vi "Get Paths Array UI.vi"(11 "Data":variant) -> (2 "Cancelled?":bool, 3 "selected_paths":string)   [LabVIEW 2019, in "LV-Data.PGSQL.lvclass"]
uses:
  LV-Data.PGSQL.lvclass
  Typedefs/Errors--enum.ctl
  <userlib>/_OpenG.lib/array/array.llb/Search 1D Array (String)__ogtk.vi
  <vilib>/regexp/Match Regular Expression.xnode
panel:
  in  "UNDO LAST VALUE":bool
  out "Paths":string[](array[string])
  out "Message":string
  out "path_to_selected_column":string="llab_038:d001(TEST_TABLE--new_stuff(hippos))"
  out "selected_table":string="TEST_TABLE"
  in  "columns_list":i32(listbox)=1
  in  "tables_list":i32(listbox)=34
  in  "STOP":bool
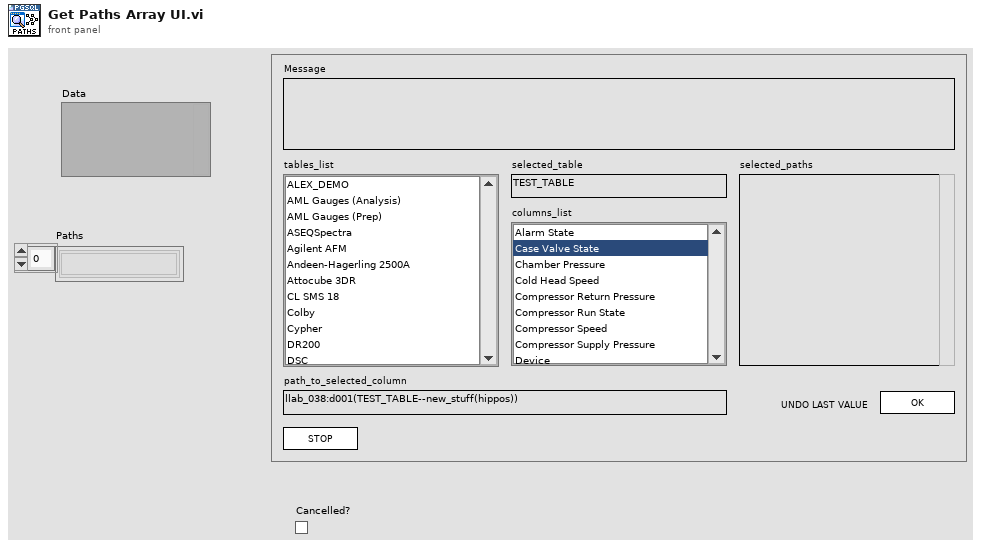
[diagram p1: front panel]
types:
  T1 = enum32{"Invalid", "Standard", "Closed", "Hidden", "Minimized", "Maximized"}
  T2 = enum32{"invalid app kind", "Development System", "Run Time System", "Student Edition", "Embedded LabVIEW", "Evaluation", "Custom"}
  T3 = enum32{"Bad", "Idle", "Run top level", "Running"}
  T4 = typedef "LV-Data.PGSQL.lvclass/Errors--enum.ctl" = enum16{"0: None", "5005: Path Type Not Supported", "5006: Number of Variables", "5007: Number of data points", "5008: Cannot write two data points", "5030: Start and End Times Identical", "5031: Input is not wholly", "5032: Undefined Timestamps", "5033: Bad path or paths", "5040: Invalid Instrument Name", "5050: Column can only hold string", "5051: Column can only hold bool", "5052: Column can only hold double", "5053: Column can only hold int"}
  T5 = cluster{"Core":cluster{"Current VI Reference":refnum<vi>, "Close Panel on Exit?":bool}, "Data.PG in":refnum<class "LV-Data.PGSQL.lvclass">, "table names":string[], "table paths":string[], "column names":string[], "column units":string[], "column paths":string[], "new table name":string, "new column name":string, "new column data type":string, "new column units":string, "selected table":string, "selected column":string, "selected table path":string, "selected column path":string, "selected column units":string, "Paths array":string[], "Current Index":i32, "Data":string[], "Type (Name)":string[]}
  T6 = cluster{"Current VI Reference":refnum<vi>, "Close Panel on Exit?":bool}
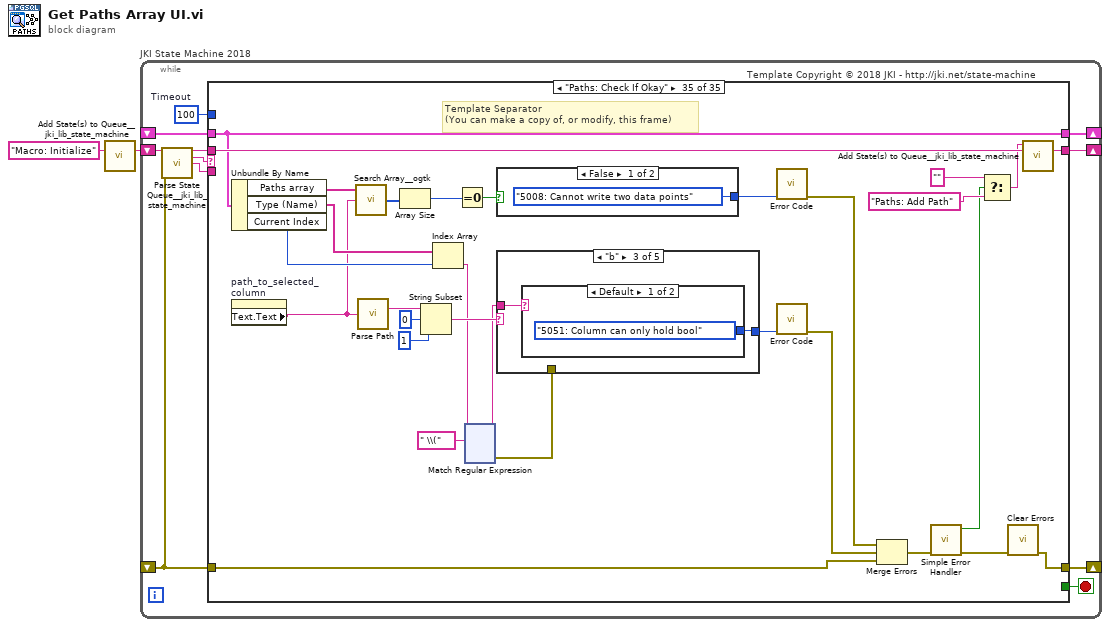
[diagram p0: block diagram]
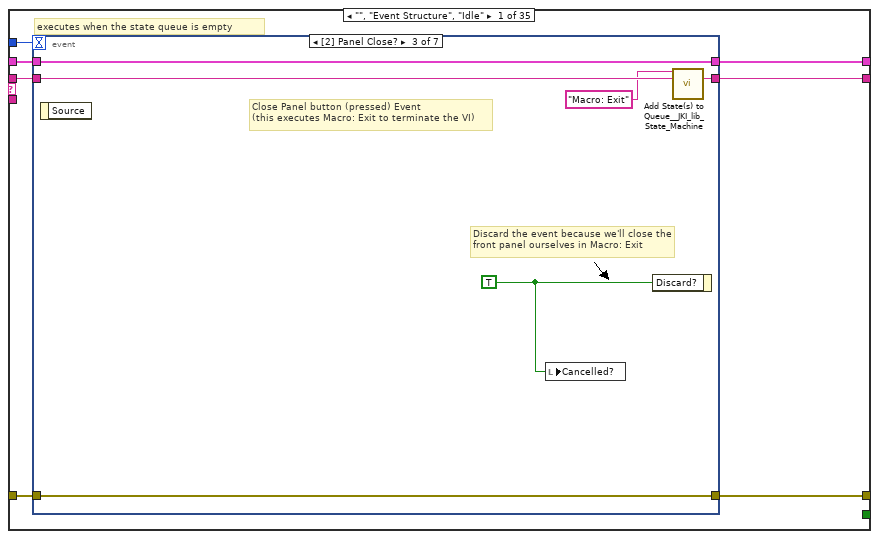
[diagram p2: hidden frame]
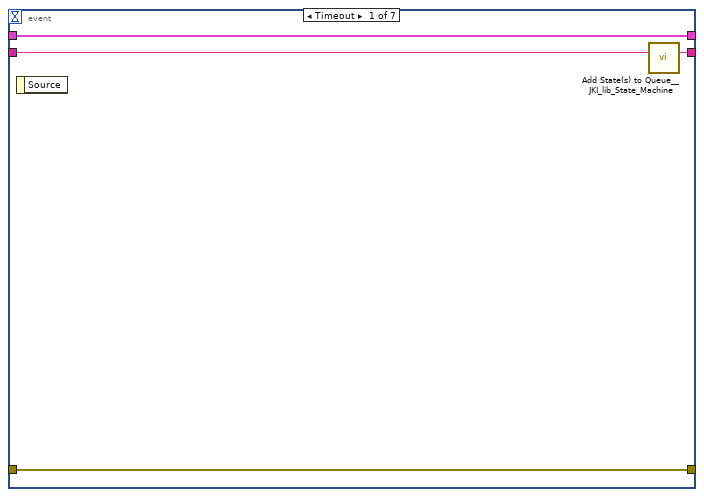
[diagram p3: hidden frame]
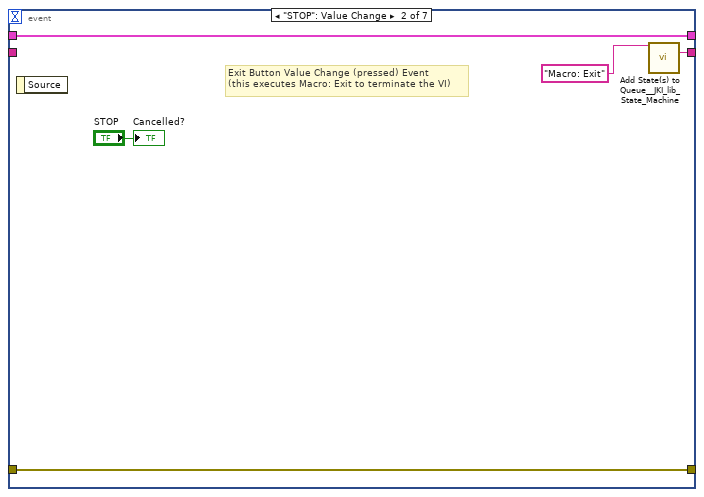
[diagram p4: hidden frame]
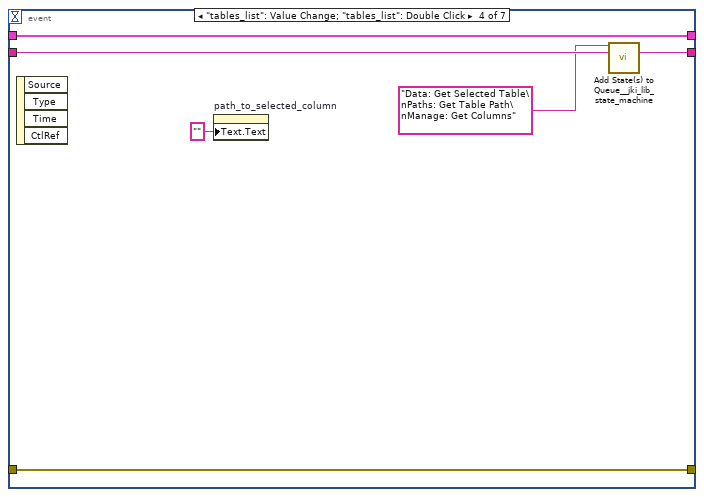
[diagram p5: hidden frame]
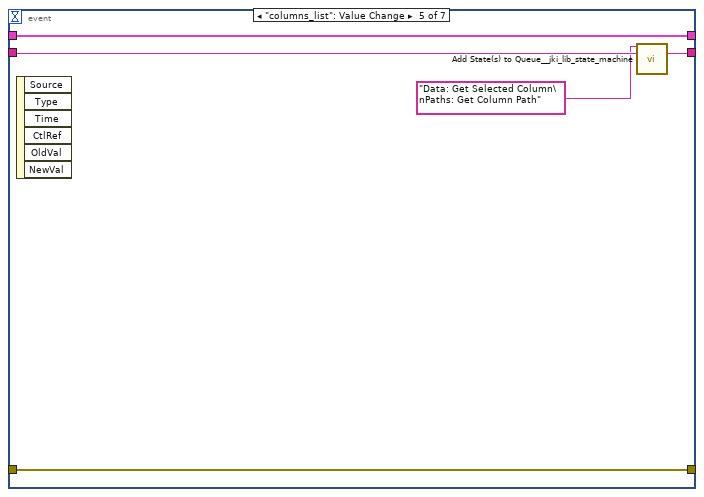
[diagram p6: hidden frame]
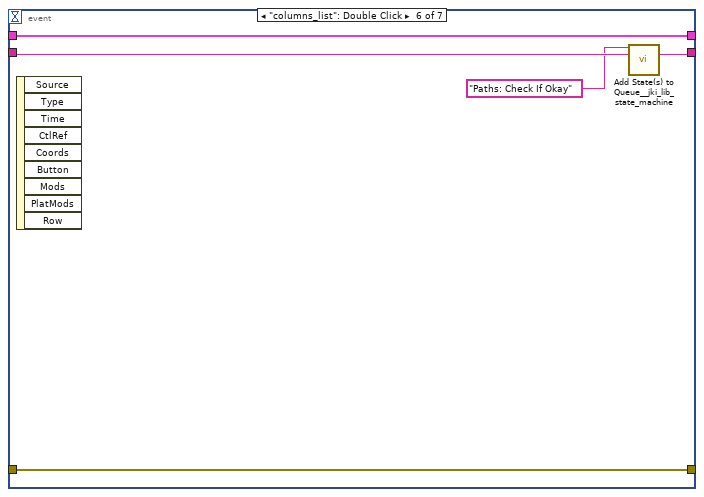
[diagram p7: hidden frame]
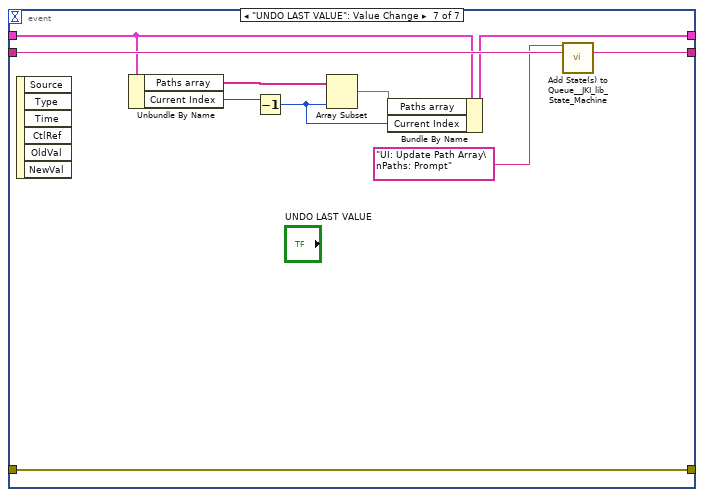
[diagram p8: hidden frame]
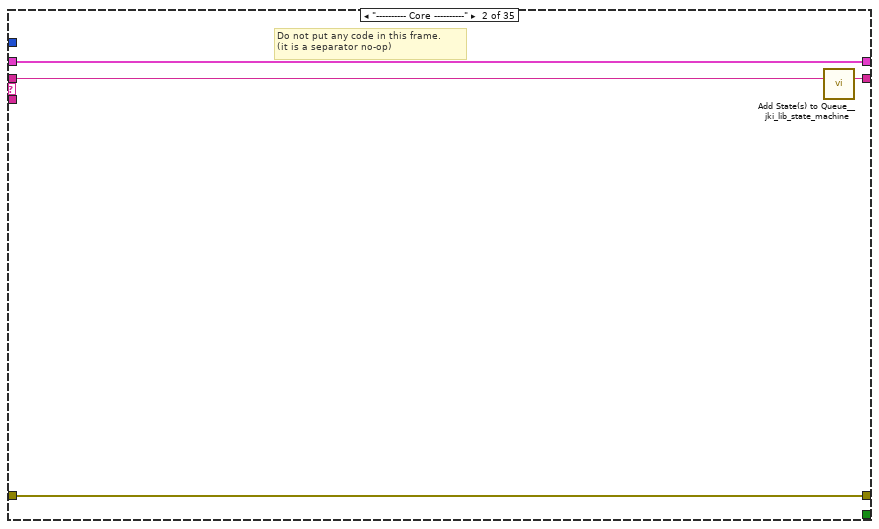
[diagram p9: hidden frame]
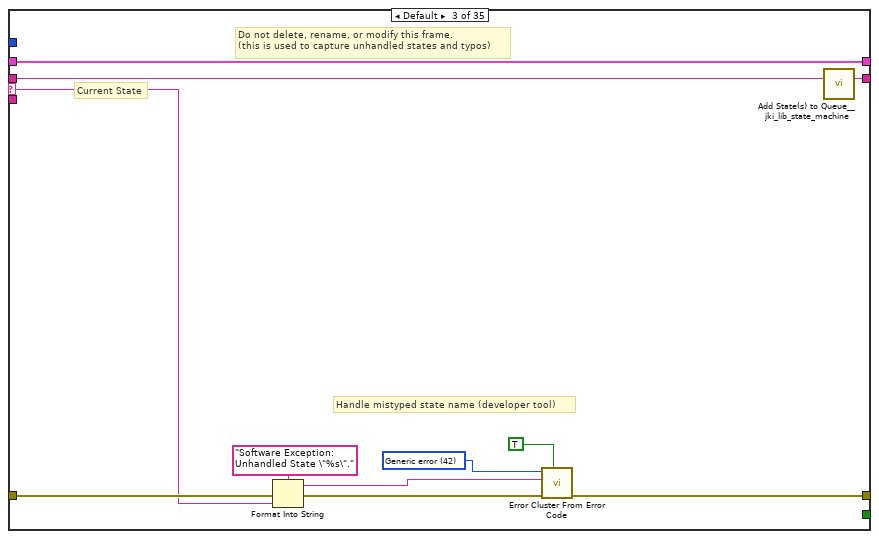
[diagram p10: hidden frame]
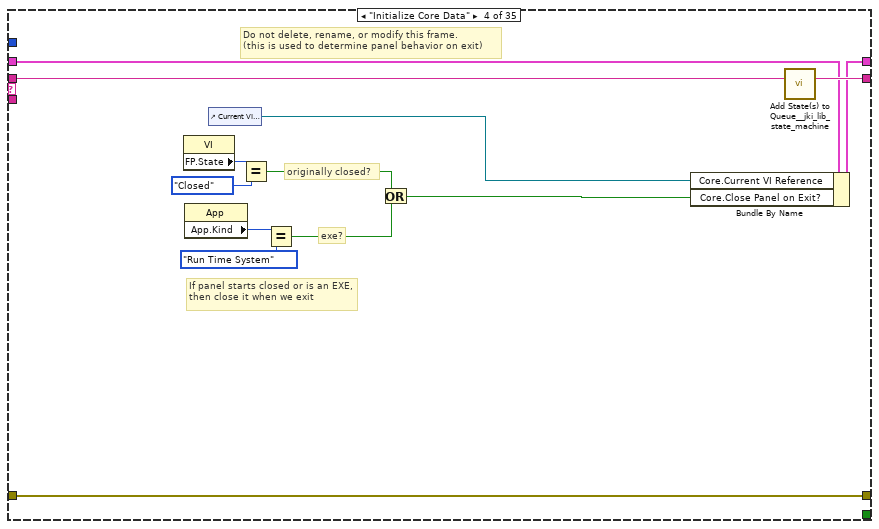
[diagram p11: hidden frame]
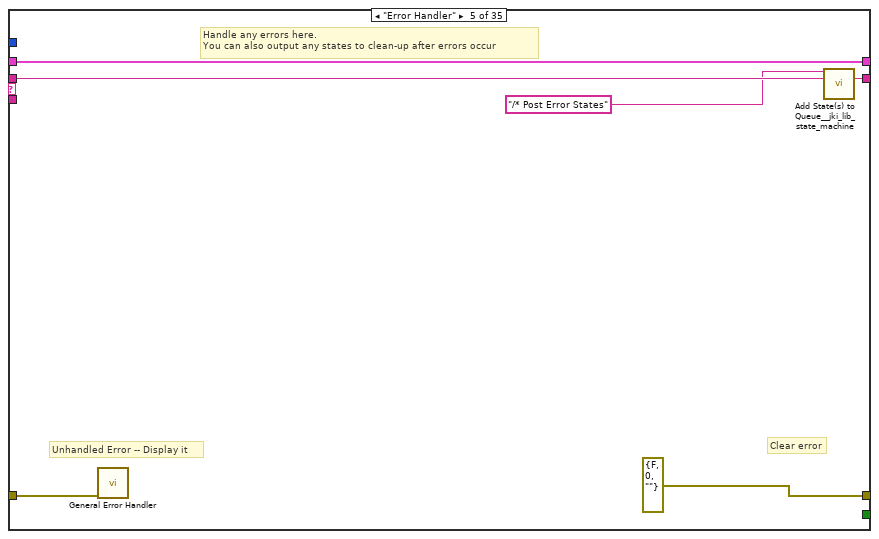
[diagram p12: hidden frame]
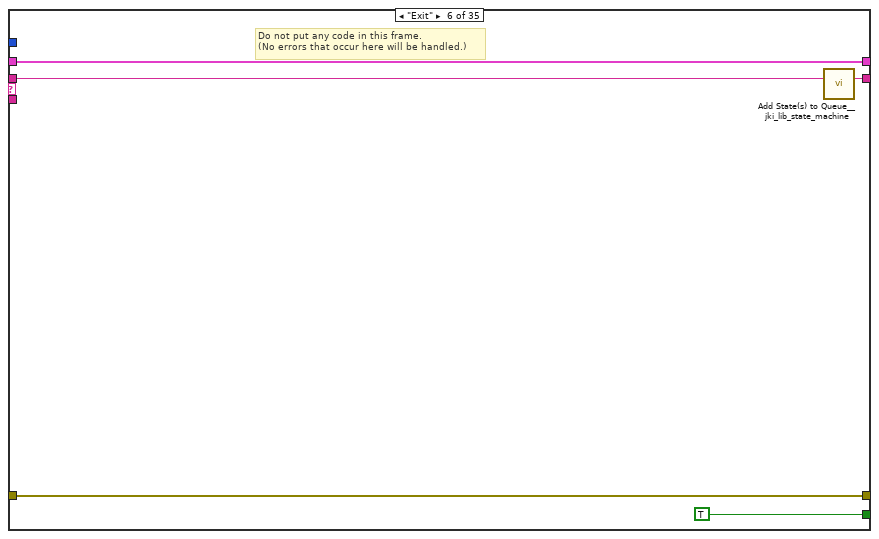
[diagram p13: hidden frame]
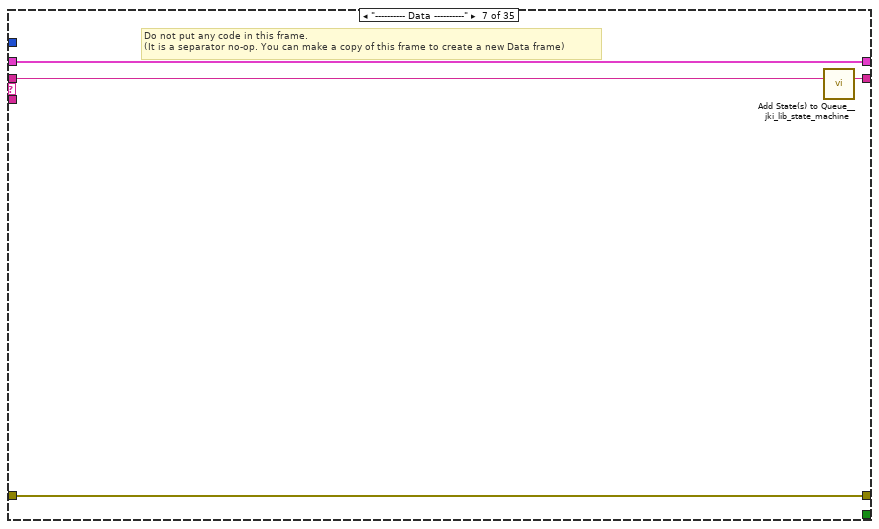
[diagram p14: hidden frame]
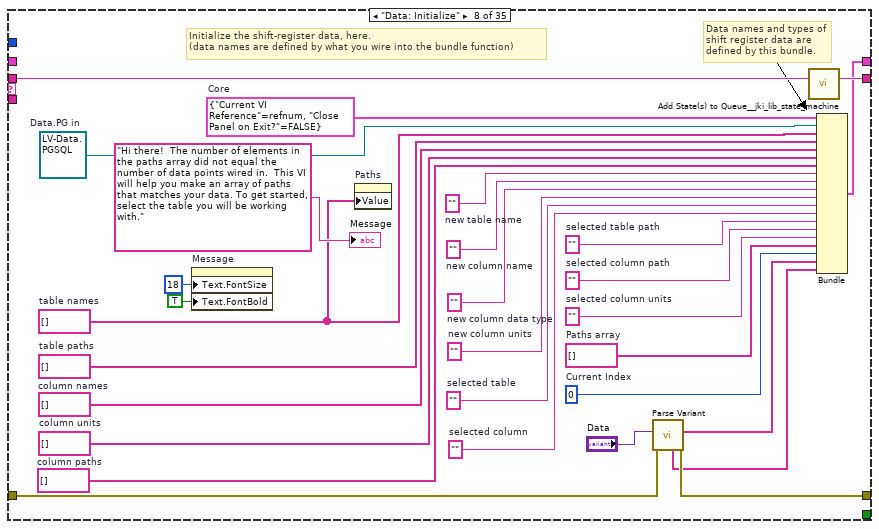
[diagram p15: hidden frame]
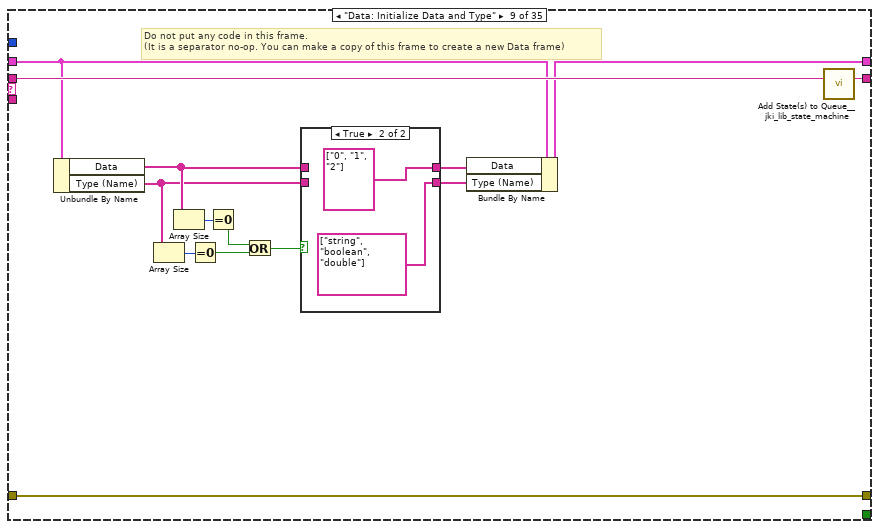
[diagram p16: hidden frame]
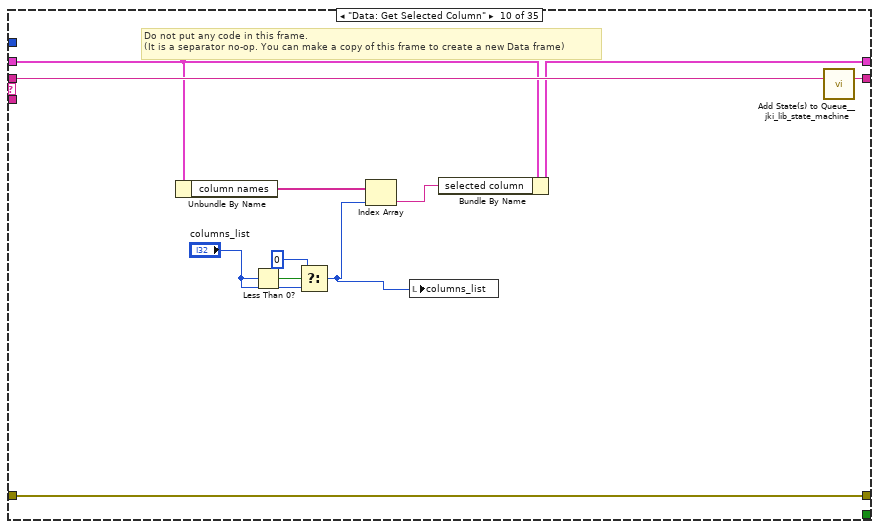
[diagram p18: hidden frame]
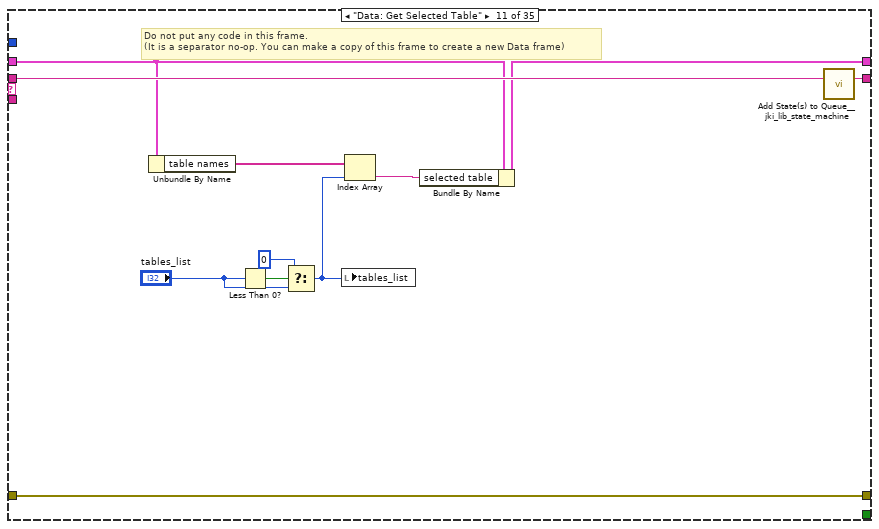
[diagram p19: hidden frame]
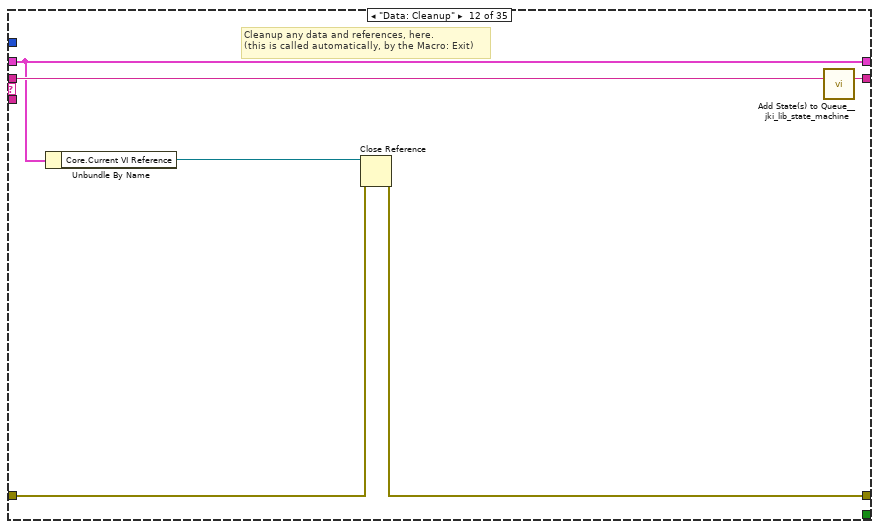
[diagram p20: hidden frame]
diagram:
  n1 = call <vilib>:"Add State(s) to Queue__jki_lib_state_machine.vi"("State(s) in (\"\")"="Macro: Initialize") -> ("States Out"=w2:string)  [unwired: 14 in]
  n2 = while "JKI State Machine 2018" {
    shift-right: [w6] -> _
    shift-left: _ -> [w5]
    shift-right: [w9] -> _
    shift-left: _ -> [w3]
    shift-right: [w8] -> _
    shift-left: w2 -> [w10]
    stop <- w7 stop-if-true
    w4 = 100  # Timeout
    # "Template Copyright © 2018 JKI - http://jki.net/state-machine"
    n3 = call <vilib>:"Parse State Queue__jki_lib_state_machine.vi"("State Queue"=w10, "Error In (no error)"=w3) -> ("Remaining States"=w12:string, "Current State"=w13:string, "Arguments"=w11:string)  [unwired: 11 in]
    n4 = case shown="\"Paths: Check If Okay\"" w13 {
      selector: w13 -> [_ _ w66 _ _ _ _ _ _ _ _ _ _ _ _ _ _ _ _ _ _ _ _ _ _ _ _ _ _ _ _ _ _ _ _]
      tunnel: w12 -> [w20 w65 w70 w89 w95 w100 w104 w133 w147 w162 w173 w179 w183 w194 w202 w208 w219 w291 w315 w323 w327 w332 w342 w346 w355 w368 w372 w378 w386 w390 w399 w413 w424 w443 w482]
      tunnel: w11 -> [_ _ _ _ _ _ _ _ _ _ _ _ _ _ _ w203 w213 _ w311 _ _ _ _ _ _ _ _ _ _ _ _ _ _ _ _]
      tunnel: w5 -> [w18 w62 w68 w82 w92 w98 w101 _ w144 w157 w168 w175 w180 w186 w197 w206 w215 w288 w312 w320 w324 w329 w339 w343 w353 w366 w369 w376 w384 w387 w397 w411 w421 w437 w480]
      tunnel: [w17 w63 w72 w86 errorcluster {"status"=FALSE, "code"=0, "source"=""} ("error out") w97 w102 w108 w145 w160 w171 w174 w181 w185 w200 w204 w216 w289 w313 w321 w325 w330 w340 w344 w349 w362 w370 w373 w380 w388 w393 w401 w422 w441 w465] -> w9
      tunnel: w3 -> [w16 w63 w71 w86 w91 w97 w102 w107 w145 w160 w171 w176 w181 w192 w200 w205 w217 w289 w313 w321 w325 w330 w340 w344 w350 w363 w370 w374 w381 w388 w394 w402 w422 w441 w462]
      tunnel: [w19 w64 w69 w88 w94 w99 w103 w132 w146 w161 w172 w178 w182 w193 w201 w207 w218 w290 w314 w322 w326 w331 w341 w345 w354 w367 w371 w377 w385 w389 w398 w412 w423 w442 w481] -> w8
      tunnel: [_ _ _ _ _ TRUE _ _ _ _ _ _ _ _ _ _ _ _ _ _ _ _ _ _ _ _ _ _ _ _ _ _ _ _ _] -> w7
      tunnel: [w15 w62 w68 w87 w92 w98 w101 w131 w143 w158 w167 w175 w180 w186 w197 w206 w215 w288 w312 w320 w324 w329 w339 w343 w352 w365 w369 w376 w383 w387 w391 w403 w421 w426 w480] -> w6
      tunnel: w4 -> [w14 _ _ _ _ _ _ _ _ _ _ _ _ _ _ _ _ _ _ _ _ _ _ _ _ _ _ _ _ _ _ _ _ _ _]
      frame "", "Event Structure", "Idle" {
        # "executes when the state queue is empty"
        n5 = event shown="[2] Panel Close?" {
          selector: _ -> [_ _ _ _ _ _ _]
          dyn-events: _ -> [_ _ _ _ _ _ _]
          timeout: w14 -> [_ _ _ _ _ _ _]
          tunnel: w20 -> [w24 _ w35 w39 w44 w49 w59]
          tunnel: [w23 w29 w34 w40 w45 w50 w60] -> w19
          tunnel: w18 -> [w21 w27 w32 w36 w46 w48 w56]
          tunnel: [w22 w28 w33 w41 w42 w51 w61] -> w17
          tunnel: w16 -> [w22 w28 w33 w41 w42 w51 w61]
          tunnel: [w21 w27 w32 w36 w46 w48 w55] -> w15
          event Timeout {
            n6 = event-data() -> ()  [unwired: 1 in, 1 out]
            n7 = call <vilib>:"Add State(s) to Queue__JKI_lib_State_Machine.vi"("State(s) in (\"\")"=w24) -> ("States Out"=w23:string)  [unwired: 14 in]
          }
          event "STOP": Value Change {
            # "Exit Button Value Change (pressed) Event\n(this executes Macro: Exit to terminate the VI)"
            n8 = event-data() -> ()  [unwired: 1 in, 1 out]
            n9 = call <vilib>:"Add State(s) to Queue__JKI_lib_State_Machine.vi"("State(s) in Front (\"\")"="Macro: Exit") -> ("States Out"=w29:string)  [unwired: 14 in]
            "Cancelled?" <- "STOP"
          }
          event Panel Close? {
            w30 = TRUE ("Discard?")
            # "Discard the event because we'll close the front panel ourselves in Macro: Exit"
            # "Close Panel button (pressed) Event\n(this executes Macro: Exit to terminate the VI)"
            n10 = event-data() -> ()  [unwired: 1 in, 1 out]
            n11 = local write "Cancelled?"(w30) -> ()
            n12 = event-data("Discard?"=w30) -> ()  [unwired: 1 in, 1 out]
            n13 = call <vilib>:"Add State(s) to Queue__JKI_lib_State_Machine.vi"("State(s) in Front (\"\")"="Macro: Exit", "State(s) in (\"\")"=w35) -> ("States Out"=w34:string)  [unwired: 13 in]
          }
          event "tables_list": Value Change; "tables_list": Double Click {
            n14 = event-data() -> ()  [unwired: 1 in, 4 out]
            n15 = property on="path_to_selected_column" class="Str"("Text.Text"="") -> ()  [unwired: 2 in, 2 out]
            n16 = call <vilib>:"Add State(s) to Queue__jki_lib_state_machine.vi"("State(s) in Front (\"\")"="Data: Get Selected Table\nPaths: Get Table Path\nManage: Get Columns" ("State(s) in Front (\"\")"), "State(s) in (\"\")"=w39) -> ("States Out"=w40:string)  [unwired: 13 in]
          }
          event "columns_list": Value Change {
            n17 = event-data() -> ()  [unwired: 1 in, 6 out]
            n18 = call <vilib>:"Add State(s) to Queue__jki_lib_state_machine.vi"("State(s) in Front (\"\")"="Data: Get Selected Column\nPaths: Get Column Path", "State(s) in (\"\")"=w44) -> ("States Out"=w45:string)  [unwired: 13 in]
          }
          event "columns_list": Double Click {
            n19 = event-data() -> ()  [unwired: 1 in, 9 out]
            n20 = call <vilib>:"Add State(s) to Queue__jki_lib_state_machine.vi"("State(s) in Front (\"\")"="Paths: Check If Okay" ("State(s) in Front (\"\")"), "State(s) in (\"\")"=w49) -> ("States Out"=w50:string)  [unwired: 13 in]
          }
          event "UNDO LAST VALUE": Value Change {
            n21 = event-data() -> ()  [unwired: 1 in, 6 out]
            n22 = Unbundle By Name(w56) -> ("Paths array"=w57:string[], "Current Index"=w58:i32)
            n23 = Decrement(x=w58) -> (x-1=w54:i32)
            n24 = Array Subset(array=w57, length=w54) -> (w53:string[])  [unwired: 1 in]
            n25 = Bundle By Name(cluster=w56, "Paths array"=w53, "Current Index"=w54) -> (w55:T5)
            n26 = call <vilib>:"Add State(s) to Queue__JKI_lib_State_Machine.vi"("State(s) in Front (\"\")"="UI: Update Path Array\nPaths: Prompt" ("State(s) in Front (\"\")"), "State(s) in (\"\")"=w59) -> ("States Out"=w60:string)  [unwired: 13 in]
          }
        }
      }
      frame "---------- Core ----------" {
        # "Do not put any code in this frame.\n(it is a separator no-op)"
        n27 = call <vilib>:"Add State(s) to Queue__jki_lib_state_machine.vi"("State(s) in (\"\")"=w65) -> ("States Out"=w64:string)  [unwired: 14 in]
      }
      frame Default {
        w75 = 42 items=["No error", "Argument error", "Memory is full", "Out of zone", "End of file", "File already open", "Generic file I/O error", "File not found", "File permission error", "Disk is full", "Duplicate path", "Too many files open", "System feature not enabled", "Resource file not found", "Cannot add resource", "Resource not found", "Image not found", "Image memory error", "Pen does not exist", "Config type invalid", "Config token not found", "Config parse error", "Config memory error", "Bad external code format", "Bad external code offset", "External code not present", "Null window", "Destroy window error", "Null menu", "Print aborted", "Bad print record", "Print driver error", "Windows error during printing", "Memory error during printing", "Print dialog error", "Generic print error", "Invalid device refnum", "Device not found", "Device parameter error", "Device unit error", "Cannot open device", "Device call aborted", "Generic error", "Cancelled by user", "Object ID too low", "Object ID too high", "Object not in heap", "Unknown heap", "Unknown object (invalid DefProc)", "Unknown object (DefProc not in table)", "Message out of range", "Invalid (null) method", "Unknown message", "Manager call not supported", "Bad address", "Network operation in progress", "Network operation timed out", "Connection is busy", "Network attribute not supported", "Network error", "Address in use", "System out of memory", "Connection aborted", "Connection refused", "Not connected", "Already connected", "Connection closed", "Initialization error (interapplication manager)", "Bad occurrence", "Wait on unbound occurrence handler", "Occurrence queue overflow", "Datalog type conflict", "Unused", "Unrecognized type (interapplication manager)", "Memory corrupt", "Failed to make temporary DLL", "Old CIN version", "Drag socket not found", "Failed to load drop-object", "Failed to register OLE object", "Failed to release OLE object", "Format specifier type mismatch", "Unknown format specifier", "Too few format specifiers", "Too many format specifiers", "Scan failed", "Newer CIN version", "Error converting to variant", "Runtime menu error", "Password tampered", "Variant attribute not found", "Incompatible variant data type", "Event data is not available", "Event Store is not present", "Occurrence is not found", "Event Queue is not created", "Event info is not available", "Refnum passed is NULL", "Error retrieving Class GUID", "Error retrieving CoClass GUID", "Error retrieving TypeLib GUID.", "Bad built application magic bytes.", "Specific driver is different from the specific driver associated with the Logical Name.", "There is no session opened to the class driver.", "Max Error", "MAX - Error with config objects", "MAX - Error loading configuration", "MAX - Group not supported"]
        # "Current State"
        # "Do not delete, rename, or modify this frame.\n(this is used to capture unhandled states and typos)"
        # "Handle mistyped state name (developer tool)"
        n28 = Format Into String(format string="Software Exception: Unhandled State \"%s\"." ("message"), error in=w71, w66) -> (resulting string=w74:string, error out=w73:errorcluster)  [unwired: 1 in]
        n29 = call <vilib>:"Error Cluster From Error Code.vi"("show call chain? (False)"=TRUE, "error in (no error)"=w73, "error message (\"\")"=w74, "error code (0)"=w75) -> ("error out"=w72:errorcluster)  [unwired: 5 in]
        n30 = call <vilib>:"Add State(s) to Queue__jki_lib_state_machine.vi"("State(s) in (\"\")"=w70) -> ("States Out"=w69:string)  [unwired: 14 in]
      }
      frame "Initialize Core Data" {
        # "Do not delete, rename, or modify this frame.\n(this is used to determine panel behavior on exit)"
        # "originally closed?"
        # "exe?"
        # "If panel starts closed or is an EXE, then close it when we exit"
        n31 = property class="VI"() -> ("FP.State"=w79:T1)  [unwired: 2 in, 2 out]
        n32 = property class="App"() -> ("App.Kind"=w85:T2)  [unwired: 2 in, 2 out]
        n33 = control-ref of="Current VI Reference"() -> (w80:refnum<vi>)
        n34 = Equal?(x=w79, y=T1."Closed" ("Front Panel Window:State")) -> (x = y?=w77:bool)
        n35 = Equal?(x=w85, y=T2."Run Time System" ("Application:Kind")) -> (x = y?=w83:bool)
        n36 = Or(x=w77, y=w83) -> (x .or. y?=w81:bool)
        n37 = Bundle By Name(cluster=w82, "Core.Current VI Reference"=w80, "Core.Close Panel on Exit?"=w81) -> (w87:T5)
        n38 = call <vilib>:"Add State(s) to Queue__jki_lib_state_machine.vi"("State(s) in (\"\")"=w89) -> ("States Out"=w88:string)  [unwired: 14 in]
      }
      frame "Error Handler" {
        # "Unhandled Error -- Display it"
        # "Handle any errors here.\nYou can also output any states to clean-up after errors occur"
        # "Clear error"
        n39 = call <vilib>:"General Error Handler.vi"("error in (no error)"=w91) -> ()  [unwired: 10 in, 5 out]
        n40 = call <vilib>:"Add State(s) to Queue__jki_lib_state_machine.vi"("State(s) in Front (\"\")"="/* Post Error States", "State(s) in (\"\")"=w95) -> ("States Out"=w94:string)  [unwired: 13 in]
      }
      frame "Exit" {
        # "Do not put any code in this frame.\n(No errors that occur here will be handled.)"
        n41 = call <vilib>:"Add State(s) to Queue__jki_lib_state_machine.vi"("State(s) in (\"\")"=w100) -> ("States Out"=w99:string)  [unwired: 14 in]
      }
      frame "---------- Data ----------" {
        # "Do not put any code in this frame.\n(It is a separator no-op. You can make a copy of this frame to create a new Data frame)"
        n42 = call <vilib>:"Add State(s) to Queue__jki_lib_state_machine.vi"("State(s) in (\"\")"=w104) -> ("States Out"=w103:string)  [unwired: 14 in]
      }
      frame "Data: Initialize" {
        w115 = 0  # Current Index
        w116 = string[] []  # Paths array
        w117 = ""  # selected column units
        w110 = ""  # selected column path
        w118 = ""  # selected table path
        w119 = ""  # selected column
        w120 = ""  # selected table
        w121 = ""  # new column units
        w122 = ""  # new column data type
        w123 = ""  # new column name
        w124 = ""  # new table name
        w125 = string[] []  # column paths
        w126 = string[] []  # column units
        w127 = string[] []  # column names
        w128 = string[] []  # table paths
        w111 = string[] []  # table names
        w129 = refnum<class "LV-Data.PGSQL.lvclass"> refnum  # Data.PG in
        w130 = T6 {"Current VI Reference"=refnum, "Close Panel on Exit?"=FALSE}  # Core
        # "Data names and types of shift register data are defined by this bundle."
        # "Initialize the shift-register data, here.\n(data names are defined by what you wire into the bundle function)"
        n43 = property on="Message" class="Str"("Text.FontSize"=u32 18 ("Text.Font:Size"), "Text.FontBold"=TRUE ("Text.Font:Bold")) -> ()  [unwired: 2 in, 2 out]
        n44 = property on="Paths" class="Arr (strict)"("Value"=w111) -> ()  [unwired: 2 in, 2 out]
        n45 = call "Parse Variant.vi"("error in"=w107, "Data"="Data") -> ("error out"=w108:errorcluster, "Data"=w109:string[], "Type (Name)"=w106:string[])  [unwired: 5 in, 2 out]
        n46 = call <vilib>:"Add State(s) to Queue__jki_lib_state_machine.vi"("State(s) in (\"\")"=w133) -> ("States Out"=w132:string)  [unwired: 14 in]
        n47 = Bundle("Core"=w130, "Data.PG in"=w129, "table names"=w111, "table paths"=w128, "column names"=w127, "column units"=w126, "column paths"=w125, "new table name"=w124, "new column name"=w123, "new column data type"=w122, "new column units"=w121, "selected table"=w120, "selected column"=w119, "selected table path"=w118, "selected column path"=w110, "selected column units"=w117, "Paths array"=w116, "Current Index"=w115, "Data"=w109, "Type (Name)"=w106) -> (w131:T5)  [unwired: 1 in]
        "Message" <- "Hi there!  The number of elements in the paths array did not equal the number of data points wired in.  This VI will help you make an array of paths that matches your data. To get started, select the table you will be working with." ("String")
      }
      frame "Data: Initialize Data and Type" {
        # "Do not put any code in this frame.\n(It is a separator no-op. You can make a copy of this frame to create a new Data frame)"
        n48 = Unbundle By Name(w144) -> ("Data"=w136:string[], "Type (Name)"=w134:string[])
        n49 = Array Size(array=w134) -> (size(s)=w141:i32)
        n50 = Array Size(array=w136) -> (size(s)=w142:i32)
        n51 = Equal To 0?(x=w141) -> (x = 0?=w139:bool)
        n52 = Equal To 0?(x=w142) -> (x = 0?=w140:bool)
        n53 = Or(x=w140, y=w139) -> (x .or. y?=w138:bool)
        n54 = case shown="True" w138 {
          tunnel: [w149 string[] ["0", "1", "2"] ("Data")] -> w137
          tunnel: w136 -> [w149 _]
          tunnel: [w148 string[] ["string", "boolean", "double"] ("Types (string)")] -> w135
          tunnel: w134 -> [w148 _]
          frame False {
          }
          frame True {
          }
        }
        n55 = Bundle By Name(cluster=w144, "Data"=w137, "Type (Name)"=w135) -> (w143:T5)
        n56 = call <vilib>:"Add State(s) to Queue__jki_lib_state_machine.vi"("State(s) in (\"\")"=w147) -> ("States Out"=w146:string)  [unwired: 14 in]
      }
      frame "Data: Get Selected Column" {
        # "Do not put any code in this frame.\n(It is a separator no-op. You can make a copy of this frame to create a new Data frame)"
        n57 = Unbundle By Name(w157) -> ("column names"=w159:string[])
        n58 = Less Than 0?(x="columns_list") -> (x < 0?=w155:bool)
        n59 = Select(t=0, s=w155, f="columns_list") -> (s? t:f=w152:i32)
        n60 = Index Array(array=w159, index=w152) -> (element=w153:string)
        n61 = local write "columns_list"(w152) -> ()
        n62 = Bundle By Name(cluster=w157, "selected column"=w153) -> (w158:T5)
        n63 = call <vilib>:"Add State(s) to Queue__jki_lib_state_machine.vi"("State(s) in (\"\")"=w162) -> ("States Out"=w161:string)  [unwired: 14 in]
      }
      frame "Data: Get Selected Table" {
        # "Do not put any code in this frame.\n(It is a separator no-op. You can make a copy of this frame to create a new Data frame)"
        n64 = Unbundle By Name(w168) -> ("table names"=w169:string[])
        n65 = Less Than 0?(x="tables_list") -> (x < 0?=w165:bool)
        n66 = Select(t=0, s=w165, f="tables_list") -> (s? t:f=w163:i32)
        n67 = local write "tables_list"(w163) -> ()
        n68 = Index Array(array=w169, index=w163) -> (element=w170:string)
        n69 = Bundle By Name(cluster=w168, "selected table"=w170) -> (w167:T5)
        n70 = call <vilib>:"Add State(s) to Queue__jki_lib_state_machine.vi"("State(s) in (\"\")"=w173) -> ("States Out"=w172:string)  [unwired: 14 in]
      }
      frame "Data: Cleanup" {
        # "Cleanup any data and references, here.\n(this is called automatically, by the Macro: Exit)"
        n71 = Unbundle By Name(w175) -> ("Core.Current VI Reference"=w177:refnum<vi>)
        n72 = Close Reference(reference=w177, error in (no error)=w176) -> (error out=w174:errorcluster)
        n73 = call <vilib>:"Add State(s) to Queue__jki_lib_state_machine.vi"("State(s) in (\"\")"=w179) -> ("States Out"=w178:string)  [unwired: 14 in]
      }
      frame "---------- UI ----------" {
        # "Do not put any code in this frame.\n(It is a separator no-op. You can make a copy of this frame to create a new UI frame)"
        n74 = call <vilib>:"Add State(s) to Queue__jki_lib_state_machine.vi"("State(s) in (\"\")"=w183) -> ("States Out"=w182:string)  [unwired: 14 in]
      }
      frame "UI: Initialize" {
        w184 = "" ("Text.Text")
        # "Initialize the User Interface, here.\n(this is called automatically, by the Macro: Init)"
        n75 = Unbundle By Name(w186) -> ("table names"=w191:string[], "column names"=w190:string[], "selected table"=→"selected_table":string)
        n76 = call <userlib>:"Fit VI window to Largest Dec__ogtk.vi"("error in (no error)"=w192) -> ("error out"=w185:errorcluster)  [unwired: 5 in, 1 out]
        n77 = property on="tables_list" class="LstBox (strict)"("Item Names"=w191) -> ()  [unwired: 2 in, 2 out]
        n78 = Build Array(0) -> (w187:i32[])
        n79 = property on="path_to_selected_column" class="Str"("Text.Text"=w184) -> ()  [unwired: 2 in, 2 out]
        n80 = local write "selected_paths"(w184) -> ()
        n81 = property on="Paths" class="Arr (strict)"("Index Values"=w187) -> ()  [unwired: 2 in, 2 out]
        n82 = property on="columns_list" class="LstBox (strict)"("Item Names"=w190) -> ()  [unwired: 2 in, 2 out]
        n83 = call <vilib>:"Add State(s) to Queue__jki_lib_state_machine.vi"("State(s) in (\"\")"=w194) -> ("States Out"=w193:string)  [unwired: 14 in]
      }
      frame "UI: Update" {
        # "Initialize the User Interface, here.\n(this is called automatically, by the Macro: Init)"
        n84 = Unbundle By Name(w197) -> ("table names"=w199:string[], "column names"=w198:string[], "selected table"=w195:string, "selected column"=w196:string)
        n85 = local write "selected_table"(w195) -> ()
        n86 = property on="tables_list" class="LstBox (strict)"("Item Names"=w199) -> ()  [unwired: 2 in, 2 out]
        n87 = property on="path_to_selected_column" class="Str"("Text.Text"=w196) -> ()  [unwired: 2 in, 2 out]
        n88 = property on="columns_list" class="LstBox (strict)"("Item Names"=w198) -> ()  [unwired: 2 in, 2 out]
        n89 = call <vilib>:"Add State(s) to Queue__jki_lib_state_machine.vi"("State(s) in (\"\")"=w202) -> ("States Out"=w201:string)  [unwired: 14 in]
      }
      frame "UI: Cursor Set" {
        # "Argument"
        # "Set and Unset Cursor Busy.\n(Usage: \"UI: Cursor Set >> Busy|Idle\")"
        n90 = case shown="\"Idle\", Default" w203 {
          tunnel: w205 -> [w210 w212]
          tunnel: [w209 w211] -> w204
          frame "Idle", Default {
            n91 = call <vilib>:"Unset Busy.vi"("error in (no error)"=w210) -> ("error out"=w209:errorcluster)  [unwired: 10 in]
          }
          frame "Busy" {
            n92 = call <vilib>:"Set Busy.vi"("error in (no error)"=w212) -> ("error out"=w211:errorcluster)  [unwired: 9 in, 1 out]
          }
        }
        n93 = call <vilib>:"Add State(s) to Queue__jki_lib_state_machine.vi"("State(s) in (\"\")"=w208) -> ("States Out"=w207:string)  [unwired: 14 in]
      }
      frame "UI: Front Panel State" {
        # "Argument"
        # "Set Front Panel Open or Closed\n(Usage: \"UI: Front Panel State >> Open|Close\")"
        n94 = Unbundle By Name(w215) -> ("Core.Current VI Reference"=w214:refnum<vi>)
        n95 = case shown="\"Maximize\", \"Maximized\"" w213 {
          tunnel: w217 -> [w225 w240 w251 w264 w277]
          tunnel: [w227 w241 w253 w266 w279] -> w216
          tunnel: w214 -> [w226 w238 w252 w265 w278]
          frame "Open", "Standard", Default {
            w220 = T1."Standard" ("State")
            n96 = property class="VI"(reference=w226, error in=w225) -> (reference out=w223:refnum<vi>, error out=w224:errorcluster, "FP.State"=w222:T1)
            n97 = Not Equal?(x=w222, y=w220) -> (x != y?=w221:bool)
            n98 = case shown="True" w221 {
              tunnel: [w231 w233] -> w227
              tunnel: w224 -> [w230 w233]
              tunnel: w223 -> [w229 _]
              tunnel: w220 -> [w228 _]
              frame True {
                n99 = invoke class="VI" method="FP.Open"(reference=w229, error in=w230, "Activate"=TRUE, "State"=w228) -> (error out=w231:errorcluster)  [unwired: 1 in, 4 out]
              }
              frame False {
              }
            }
          }
          frame "Close", "Closed" {
            n100 = property class="VI"(reference=w238, error in=w240) -> (reference out=w237:refnum<vi>, error out=w239:errorcluster, "FP.State"=w235:T1)
            n101 = Not Equal?(x=w235, y=T1."Closed" ("Front Panel Window:State")) -> (x != y?=w234:bool)
            n102 = case shown="True" w234 {
              tunnel: [w242 w245] -> w241
              tunnel: w239 -> [w242 w244]
              tunnel: w237 -> [_ w243]
              frame False {
              }
              frame True {
                n103 = invoke class="VI" method="FP.Close"(reference=w243, error in=w244) -> (error out=w245:errorcluster)  [unwired: 1 in, 2 out]
              }
            }
          }
          frame "Hidden", "Hide" {
            w246 = T1."Hidden" ("State")
            n104 = property class="VI"(reference=w252, error in=w251) -> (reference out=w249:refnum<vi>, error out=w250:errorcluster, "FP.State"=w248:T1)
            n105 = Not Equal?(x=w248, y=w246) -> (x != y?=w247:bool)
            n106 = case shown="True" w247 {
              tunnel: [w257 w258] -> w253
              tunnel: w250 -> [w256 w258]
              tunnel: w249 -> [w255 _]
              tunnel: w246 -> [w254 _]
              frame True {
                n107 = invoke class="VI" method="FP.Open"(reference=w255, error in=w256, "State"=w254) -> (error out=w257:errorcluster)  [unwired: 2 in, 4 out]
              }
              frame False {
              }
            }
          }
          frame "Minimize", "Minimized" {
            w259 = T1."Minimized" ("State")
            n108 = property class="VI"(reference=w265, error in=w264) -> (reference out=w262:refnum<vi>, error out=w263:errorcluster, "FP.State"=w261:T1)
            n109 = Not Equal?(x=w261, y=w259) -> (x != y?=w260:bool)
            n110 = case shown="True" w260 {
              tunnel: [w270 w271] -> w266
              tunnel: w263 -> [w269 w271]
              tunnel: w262 -> [w268 _]
              tunnel: w259 -> [w267 _]
              frame True {
                n111 = invoke class="VI" method="FP.Open"(reference=w268, error in=w269, "State"=w267) -> (error out=w270:errorcluster)  [unwired: 2 in, 4 out]
              }
              frame False {
              }
            }
          }
          frame "Maximize", "Maximized" {
            w272 = T1."Maximized" ("State")
            n112 = property class="VI"(reference=w278, error in=w277) -> (reference out=w275:refnum<vi>, error out=w276:errorcluster, "FP.State"=w274:T1)
            n113 = Not Equal?(x=w274, y=w272) -> (x != y?=w273:bool)
            n114 = case shown="True" w273 {
              tunnel: [w283 w284] -> w279
              tunnel: w276 -> [w282 w284]
              tunnel: w275 -> [w281 _]
              tunnel: w272 -> [w280 _]
              frame True {
                n115 = invoke class="VI" method="FP.Open"(reference=w281, error in=w282, "State"=w280) -> (error out=w283:errorcluster)  [unwired: 2 in, 4 out]
              }
              frame False {
              }
            }
          }
        }
        n116 = call <vilib>:"Add State(s) to Queue__jki_lib_state_machine.vi"("State(s) in (\"\")"=w219) -> ("States Out"=w218:string)  [unwired: 14 in]
      }
      frame "UI: Update Path Array" {
        # "Do not put any code in this frame.\n(It is a separator no-op. You can make a copy of this frame to create a new UI frame)"
        n117 = Unbundle By Name(w288) -> ("Paths array"=w286:string[])
        "Paths" <- w286
        n118 = call <userlib>:"1D Array to String__ogtk.vi"("delimiter (Tab)"="\n", "Array of Strings"=w286) -> ("delimited string"=→"selected_paths":string)  [unwired: 9 in]
        n119 = call <vilib>:"Add State(s) to Queue__jki_lib_state_machine.vi"("State(s) in (\"\")"=w291) -> ("States Out"=w290:string)  [unwired: 14 in]
      }
      frame "UI: Wait" {
        # "Do not put any code in this frame.\n(It is a separator no-op. You can make a copy of this frame to create a new UI frame)"
        n120 = property class="VI"() -> ("Exec.State"=w297:T3)  [unwired: 2 in, 2 out]
        n121 = To Lower Case(string=w311) -> (all lower case string=w309:string)
        n122 = Equal?(x=T3."Run top level", y=w297) -> (x = y?=w295:bool)
        n123 = Equal?(x=w309, y="reset") -> (x = y?=w308:bool)
        n124 = Select(t=u32 15000 ("milliseconds to wait"), s=w295, f=u32 2000 ("milliseconds to wait")) -> (s? t:f=w293:u32)
        n125 = call <userlib>:"Periodic Trigger__ogtk.vi"("time (ms)"=w293, "reset"=w308) -> ("Triggered"=w307:bool, "timer value"=w304:u32)  [unwired: 11 in, 1 out]
        n126 = Subtract(x=w293, y=w304) -> (x-y=w302:u32)
        n127 = Divide(x=w302, y=u32 1000) -> (x/y=w298:dbl)
        n128 = Select(t="Macro: Exit" ("y"), s=w307, f="Idle\nUI: Wait" ("y")) -> (s? t:f=w300:string)
        n129 = Format Into String(format string="Great work! Your paths have been copied to your clipboard.  Find where you placed Insert.vi, wire a string constant to the control for paths, and paste the text from your clipboard into the string constant.  This VI will close after %d seconds " ("Text.Text"), w298) -> (resulting string=w301:string)  [unwired: 2 in, 1 out]
        n130 = property on="Message" class="Str"("Text.Text"=w301) -> ()  [unwired: 2 in, 2 out]
        n131 = call <vilib>:"Add State(s) to Queue__jki_lib_state_machine.vi"("State(s) in (\"\")"=w315, "State(s) at Back (\"\")"=w300) -> ("States Out"=w314:string)  [unwired: 13 in]
      }
      frame "UI: Finish" {
        # "Do not put any code in this frame.\n(It is a separator no-op. You can make a copy of this frame to create a new UI frame)"
        n132 = Unbundle By Name(w320) -> ("Paths array"=w319:string[])
        n133 = call <userlib>:"1D Array to String__ogtk.vi"("delimiter (Tab)"="\n", "Array of Strings"=w319) -> ("delimited string"=w318:string)  [unwired: 9 in]
        n134 = invoke class="App" method="Clipboard.Write"("Param 0"=w318) -> ()  [unwired: 3 in, 4 out]
        n135 = call <vilib>:"Add State(s) to Queue__jki_lib_state_machine.vi"("State(s) in Front (\"\")"="" ("State(s) in Front (\"\")"), "State(s) in (\"\")"=w323) -> ("States Out"=w322:string)  [unwired: 13 in]
      }
      frame "---------- Macro ----------" {
        # "Do not put any code in this frame.\n(It is a separator no-op. You can make a copy of this frame to create a new Macro frame)"
        n136 = call <vilib>:"Add State(s) to Queue__jki_lib_state_machine.vi"("State(s) in (\"\")"=w327) -> ("States Out"=w326:string)  [unwired: 14 in]
      }
      frame "Macro: Initialize" {
        w328 = "Data: Initialize\nInitialize Core Data\nUI: Initialize\nUI: Front Panel State >> Open\nData: Initialize Data and Type\n\nConnection: Open\nManage: Get Tables\nUI: Update\n\n//Data: Get Selected Table\n//Paths: Get Table Path\n\n//Manage: Get Columns\n//UI: Update\n//Data: Get Selected Column\n\n//Paths: Get Column Path"  # Data: Initialize Initialize Core Data UI: Initialize UI: Front Panel State >> Open Data: Initialize Data and Type  Connection: Open Manage: Get Tables UI: Update  //Data: Get Selected Table //Paths: Get Table Path  //Manage: Get Columns //UI: Update //Data: Get Selected Column  //Paths: Get Column Path
        # "Initialization Macro\n(This is called once, when the VI starts)"
        n137 = call <vilib>:"Add State(s) to Queue__jki_lib_state_machine.vi"("State(s) in Front (\"\")"=w328, "State(s) in (\"\")"=w332) -> ("States Out"=w331:string)  [unwired: 13 in]
      }
      frame "Macro: Exit" {
        # "Exit Macro\n(This is called once, when the VI exits)"
        n138 = Unbundle By Name(w339) -> ("Core.Close Panel on Exit?"=w338:bool)
        n139 = Select(t="UI: Front Panel State >> Close", s=w338, f="") -> (s? t:f=w335:string)
        n140 = call <vilib>:"Add State(s) to Queue__jki_lib_state_machine.vi"("State(s) in (\"\")"=w335, "State(s) at Back (\"\")"="Connection: Close\nData: Cleanup\nExit") -> ("States Out"=w333:string)  [unwired: 13 in]
        n141 = call <vilib>:"Add State(s) to Queue__jki_lib_state_machine.vi"("State(s) in Front (\"\")"=w333, "State(s) in (\"\")"=w342) -> ("States Out"=w341:string)  [unwired: 13 in]
      }
      frame "---------- Manage ----------" {
        # "Template Separator\n(You can make a copy of, or modify, this frame)"
        n142 = call <vilib>:"Add State(s) to Queue__jki_lib_state_machine.vi"("State(s) in (\"\")"=w346) -> ("States Out"=w345:string)  [unwired: 14 in]
      }
      frame "Manage: Get Tables" {
        # "Your code here.\n(You can make a copy of, or modify, this frame)"
        n143 = Unbundle By Name(w353) -> ("Data.PG in"=w351:refnum<class "LV-Data.PGSQL.lvclass">)
        n144 = call "List Tables.vi"("error in (no error)"=w350, "Data.PG"=w351) -> ("error out"=w349:errorcluster, "Table Paths"=w347:string[], "Table Names"=w348:string[])  [unwired: 6 in, 1 out]
        n145 = Bundle By Name(cluster=w353, "table names"=w348, "table paths"=w347) -> (w352:T5)
        n146 = call <vilib>:"Add State(s) to Queue__jki_lib_state_machine.vi"("State(s) in (\"\")"=w355) -> ("States Out"=w354:string)  [unwired: 14 in]
      }
      frame "Manage: Get Columns" {
        # "Your code here.\n(You can make a copy of, or modify, this frame)"
        n147 = Unbundle By Name(w366) -> ("Data.PG in"=w361:refnum<class "LV-Data.PGSQL.lvclass">, "selected table path"=w360:string)
        n148 = call "List Columns.vi"("error in (no error)"=w363, "Table Path"=w360, "Data.PG"=w361) -> ("error out"=w362:errorcluster, "Column Paths"=w357:string[], "Column Names"=w359:string[], "Data.PG out"=w358:refnum<class "LV-Data.PGSQL.lvclass">, "Column Units"=w356:string[])  [unwired: 4 in]
        n149 = Bundle By Name(cluster=w366, "Data.PG in"=w358, "column names"=w359, "column paths"=w357, "column units"=w356) -> (w365:T5)
        n150 = call <vilib>:"Add State(s) to Queue__jki_lib_state_machine.vi"("State(s) in Front (\"\")"="UI: Update\nPaths: Prompt" ("State(s) in Front (\"\")"), "State(s) in (\"\")"=w368) -> ("States Out"=w367:string)  [unwired: 13 in]
      }
      frame "---------- Connection ----------" {
        # "Template Separator\n(You can make a copy of, or modify, this frame)"
        n151 = call <vilib>:"Add State(s) to Queue__jki_lib_state_machine.vi"("State(s) in (\"\")"=w372) -> ("States Out"=w371:string)  [unwired: 14 in]
      }
      frame "Connection: Close" {
        # "Template Separator\n(You can make a copy of, or modify, this frame)"
        n152 = Unbundle By Name(w376) -> ("Data.PG in"=w375:refnum<class "LV-Data.PGSQL.lvclass">)
        n153 = call-dynamic "Close.vi"("error in (no error)"=w374, "Data.PG in"=w375) -> ("error out"=w373:errorcluster)  [unwired: 8 in, 1 out]
        n154 = call <vilib>:"Add State(s) to Queue__jki_lib_state_machine.vi"("State(s) in (\"\")"=w378) -> ("States Out"=w377:string)  [unwired: 14 in]
      }
      frame "Connection: Open" {
        # "Template Separator\n(You can make a copy of, or modify, this frame)"
        n155 = Unbundle By Name(w384) -> ("Data.PG in"=w379:refnum<class "LV-Data.PGSQL.lvclass">)
        n156 = call "PGSQL.Open.vi"("error in (no error)"=w381, "Data.PG in"=w379) -> ("error out"=w380:errorcluster, "Data.PG out"=w382:refnum<class "LV-Data.PGSQL.lvclass">)  [unwired: 8 in]
        n157 = Bundle By Name(cluster=w384, "Data.PG in"=w382) -> (w383:T5)
        n158 = call <vilib>:"Add State(s) to Queue__jki_lib_state_machine.vi"("State(s) in (\"\")"=w386) -> ("States Out"=w385:string)  [unwired: 14 in]
      }
      frame "---------- Paths ----------" {
        # "Template Separator\n(You can make a copy of, or modify, this frame)"
        n159 = call <vilib>:"Add State(s) to Queue__jki_lib_state_machine.vi"("State(s) in (\"\")"=w390) -> ("States Out"=w389:string)  [unwired: 14 in]
      }
      frame "Paths: Get Table Path" {
        # "Template Separator\n(You can make a copy of, or modify, this frame)"
        n160 = Unbundle By Name(w397) -> ("Data.PG in"=w396:refnum<class "LV-Data.PGSQL.lvclass">, "selected table"=w395:string)
        n161 = call "Get Table Path.vi"("error in (no error)"=w394, "Table Name"=w395, "Data.PG"=w396) -> ("error out"=w393:errorcluster, "Table Path"=w392:string)  [unwired: 5 in, 2 out]
        n162 = Bundle By Name(cluster=w397, "selected table path"=w392) -> (w391:T5)
        n163 = call <vilib>:"Add State(s) to Queue__jki_lib_state_machine.vi"("State(s) in (\"\")"=w399) -> ("States Out"=w398:string)  [unwired: 14 in]
      }
      frame "Paths: Get Column Path" {
        # "Template Separator\n(You can make a copy of, or modify, this frame)"
        n164 = Unbundle By Name(w411) -> ("Data.PG in"=w407:refnum<class "LV-Data.PGSQL.lvclass">, "selected table path"=w400:string, "selected column"=w406:string, "selected table"=w410:string, "selected column"=w409:string)
        n165 = call "Get Column Path.vi"("error in (no error)"=w402, "Column Name"=w406, "Table path"=w400, "Data.PG in"=w407) -> ("error out"=w401:errorcluster, "Column Unit"=w404:string, "Column Path"=w405:string)  [unwired: 4 in, 1 out]
        n166 = call "Build Path.vi"("Table path"=w400, "Column path"=w405, "Table name"=w410, "Column name"=w409, "Column units"=w404) -> ("PG path"=→"path_to_selected_column":string)  [unwired: 10 in]
        n167 = Bundle By Name(cluster=w411, "selected column path"=w405, "selected column units"=w404) -> (w403:T5)
        n168 = call <vilib>:"Add State(s) to Queue__jki_lib_state_machine.vi"("State(s) in (\"\")"=w413) -> ("States Out"=w412:string)  [unwired: 14 in]
      }
      frame "Paths: Prompt" {
        # "Template Separator\n(You can make a copy of, or modify, this frame)"
        n169 = Unbundle By Name(w421) -> ("Current Index"=w416:i32, "Type (Name)"=w418:string[], "Data"=w417:string[])
        n170 = Index Array(array=w418, index=w416) -> (element=w419:string)
        n171 = Index Array(array=w417, index=w416) -> (element=w415:string)
        n172 = Format Into String(format string="Element number --%d-- of data is of type --%s-- and has a value of --%s--.\nPlease double-click the column that stores this element", w416, w419, w415) -> (resulting string=w414:string)  [unwired: 2 in, 1 out]
        n173 = property on="Message" class="Str"("Text.Text"=w414) -> ()  [unwired: 2 in, 2 out]
        n174 = call <vilib>:"Add State(s) to Queue__jki_lib_state_machine.vi"("State(s) in (\"\")"=w424) -> ("States Out"=w423:string)  [unwired: 14 in]
      }
      frame "Paths: Add Path" {
        # "Template Separator\n(You can make a copy of, or modify, this frame)"
        n175 = Unbundle By Name(w437) -> ("Paths array"=w440:string[], "Current Index"=w435:i32, "Data"=w436:string[])
        n176 = Increment(x=w435) -> (x+1=w427:i32)
        n177 = Array Size(array=w436) -> (size(s)=w434:i32)
        n178 = Greater?(x=w427, y=4) -> (0:w431:bool)
        n179 = Equal?(x=w427, y=w434) -> (x = y?=w433:bool)
        n180 = case shown="True" w431 {
          tunnel: w427 -> [_ w447]
          tunnel: [0 w445] -> w428
          frame False {
          }
          frame True {
            n181 = Subtract(x=w447, y=4) -> (x-y=w445:i32)
          }
        }
        n182 = case shown="True" w433 {
          tunnel: w427 -> [w449 w452]
          tunnel: [w449 w451] -> w425
          tunnel: ["UI: Update Path Array\nPaths: Prompt" ("State(s) in Front (\"\")") "UI: Update Path Array\nUI: Finish\nUI: Wait >> reset" ("State(s) in Front (\"\")")] -> w432
          frame False {
          }
          frame True {
            n183 = Decrement(x=w452) -> (x-1=w451:i32)
          }
        }
        n184 = property on="path_to_selected_column" class="Str"() -> ("Text.Text"=w439:string)  [unwired: 2 in, 2 out]
        n185 = Build Array(w428) -> (w429:i32[])
        n186 = property on="Paths" class="Arr (strict)"("Index Values"=w429) -> ()  [unwired: 2 in, 2 out]
        n187 = Insert Into Array(array=w440, new element=w439) -> (w438:string[])  [unwired: 1 in]
        n188 = Bundle By Name(cluster=w437, "Paths array"=w438, "Current Index"=w425) -> (w426:T5)
        n189 = call <vilib>:"Add State(s) to Queue__jki_lib_state_machine.vi"("State(s) in Front (\"\")"=w432, "State(s) in (\"\")"=w443) -> ("States Out"=w442:string)  [unwired: 13 in]
      }
      frame "Paths: Check If Okay" {
        # "Template Separator\n(You can make a copy of, or modify, this frame)"
        n190 = Unbundle By Name(w480) -> ("Paths array"=w479:string[], "Type (Name)"=w473:string[], "Current Index"=w472:i32)
        n191 = property on="path_to_selected_column" class="Str"() -> ("Text.Text"=w464:string)  [unwired: 2 in, 2 out]
        n192 = call-poly <userlib>:"Search Array__ogtk.vi"("Array"=w479, "Element Data"=w464) -> ("Indices of Elements"=w478:i32[])  [unwired: 7 in]
        n193 = call "Parse Path.vi"("PG Path"=w464) -> ("Column path"=w463:string)  [unwired: 10 in, 4 out]
        n194 = Array Size(array=w478) -> (size(s)=w477:i32)
        n195 = String Subset(string=w463, offset (0)=0, length (rest)=1 ("length (rest)")) -> (substring=w461:string)
        n196 = Index Array(array=w473, index=w472) -> (element=w456:string)
        n197 = Equal To 0?(x=w477) -> (x = 0?=w476:bool)
        n198 = xnode "Match Regular Expression"("input string"=w456, "regular expression"=" \\(") -> ("before match"=w455:string, "error out"=w454:errorcluster)  [unwired: 4 in, 3 out]
        n199 = case shown="False" w476 {
          tunnel: [Errors--enum."5008: Cannot write two data points" ("Error code") Errors--enum."0: None" ("Error code")] -> w459
          frame False {
          }
          frame True {
          }
        }
        n200 = case shown="\"b\"" w461 {
          tunnel: w455 -> [_ w599 w603 w607 w611]
          tunnel: [Errors--enum."5005: Path Type Not Supported" ("Error code") w598 w602 w606 w610] -> w458
          tunnel: w454 -> [_ _ _ _ _]
          frame "False", Default {
          }
          frame "v" {
            n201 = case shown="Default" w599 {
              tunnel: [Errors--enum."5050: Column can only hold string" ("Error code") Errors--enum."0: None" ("Error code")] -> w598
              frame Default {
              }
              frame "string" {
              }
            }
          }
          frame "b" {
            n202 = case shown="Default" w603 {
              tunnel: [Errors--enum."5051: Column can only hold bool" ("Error code") Errors--enum."0: None" ("Error code")] -> w602
              frame Default {
              }
              frame "boolean" {
              }
            }
          }
          frame "d" {
            n203 = case shown="Default" w607 {
              tunnel: [Errors--enum."5052: Column can only hold double" ("Error code") Errors--enum."0: None" ("Error code")] -> w606
              frame Default {
              }
              frame "double", "integer" {
              }
            }
          }
          frame "i" {
            n204 = case shown="Default" w611 {
              tunnel: [Errors--enum."5053: Column can only hold int" ("Error code") Errors--enum."0: None" ("Error code")] -> w610
              frame Default {
              }
              frame "integer" {
              }
            }
          }
        }
        n205 = call "Error Code.vi"("Error code"=w459) -> ("error out"=w460:errorcluster)  [unwired: 10 in]
        n206 = call "Error Code.vi"("Error code"=w458) -> ("error out"=w457:errorcluster)  [unwired: 10 in]
        n207 = Merge Errors(w460, w457, w462) -> (w471:errorcluster)
        n208 = call <vilib>:"Simple Error Handler.vi"("error in (no error)"=w471) -> ("error?"=w468:bool, "error out"=w466:errorcluster)  [unwired: 4 in, 3 out]
        n209 = Select(t="", s=w468, f="Paths: Add Path") -> (s? t:f=w467:string)
        n210 = call <vilib>:"Clear Errors.vi"("error in (no error)"=w466) -> ("error out"=w465:errorcluster)  [unwired: 5 in, 1 out]
        n211 = call <vilib>:"Add State(s) to Queue__jki_lib_state_machine.vi"("State(s) in Front (\"\")"=w467, "State(s) in (\"\")"=w482) -> ("States Out"=w481:string)  [unwired: 13 in]
      }
    }
  }
